vi "dfd_DFXPSimu AccAdd (vector).vi"(5 "quantize output?":bool=TRUE, 7 "op params":T2={"source"=0, "is floating?"=FALSE, "o-mode"=enum."Wrap", "q-mode"=enum."Truncation", "wl"=1, "high limit"=0, "low limit"=0, "iwl"=0, "sign?"=TRUE} {"source" items=["Coef a/k"=0, "Coef b/v"=7, "Input"=1, "Output"=2, "Multiplicand"=3, "Product"=4, "Sum"=5, "Delay"=6, "Gain"=8]}, 8 "filtering statistics in":T6(array[cluster]) {"statistics information"."min value" format="%.2f"; "statistics information"."max value" format="%.2f"; "Quantizer Source" items=["Coefficients a/k"=0, "Coefficients b/v"=7, "Input"=1, "Output"=2, "Multiplicand"=3, "Product"=4, "Sum"=5, "Delay"=6]}, 10 "addends":T7, 11 "acc in":T1={"value"=0, "wl"=0, "iwl"=0, "Signed"=TRUE} {"value" format="%.0x"}) -> (0 "filtering statistics out":T6(array[cluster]) {"statistics information"."min value" format="%.2f"; "statistics information"."max value" format="%.2f"; "Quantizer Source" items=["Coefficients a/k"=0, "Coefficients b/v"=7, "Input"=1, "Output"=2, "Multiplicand"=3, "Product"=4, "Sum"=5, "Delay"=6]}, 3 "acc out":T1={"value"=0, "wl"=0, "iwl"=0, "Signed"=TRUE} {"value" format="%.0x"})   [LabVIEW 2017, in "NI_DigFilter_FXP.lvlib"]
uses:
  <vilib>/addons/Digital Filter Design/NI_DigFilter_FXP.lvlib
  <vilib>/addons/Digital Filter Design/_Objects.llb/dfd_DFXP Data Type (scaler).ctl
  <vilib>/addons/Digital Filter Design/_Objects.llb/dfd_DFXP Data Type (vector).ctl
  <vilib>/addons/Digital Filter Design/_Objects.llb/DFD Quantization Sources.ctl
  <vilib>/addons/Digital Filter Design/_Objects.llb/DFD FXP Statistics Data.ctl
  <vilib>/addons/Digital Filter Design/_Objects.llb/dfd_DFXP Operation Parameter.ctl
  <vilib>/addons/Digital Filter Design/_Objects.llb/dfd_Internal Quantization Srcs.ctl
  <vilib>/addons/Digital Filter Design/NI_DigFilterLicensed.lvlib
panel:
  in  "addend type":T1={"value"=0, "wl"=0, "iwl"=0, "Signed"=TRUE} {"value" format="%.0x"}
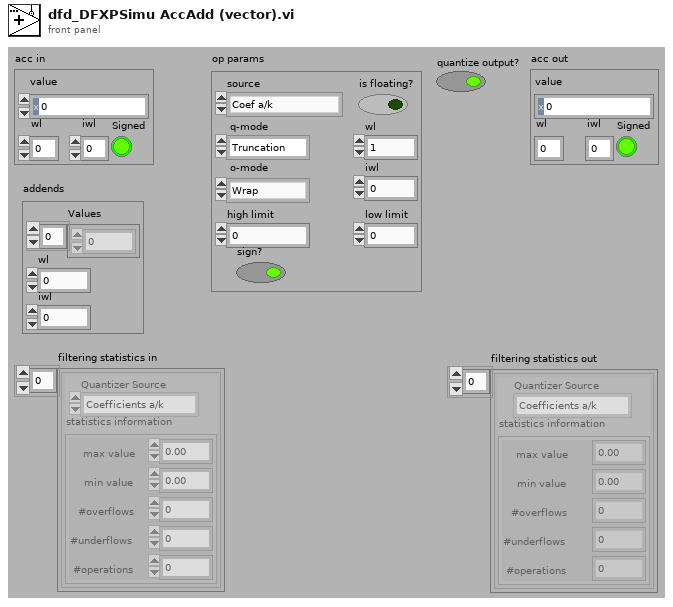
[diagram p1: front panel]
types:
  T1 = typedef "dfd_DFXP Data Type (scaler).ctl" = cluster{"value":i64, "wl":i16, "iwl":i16, "Signed":bool}
  T2 = typedef "dfd_DFXP Operation Parameter.ctl" = cluster{"source":T3, "is floating?":bool, "o-mode":enum16{"Saturation", "Wrap"}, "q-mode":enum16{"Nearest", "Truncation"}, "wl":i16, "high limit":i64, "low limit":i64, "iwl":i16, "sign?":bool}
  T3 = typedef "NI_DigFilterLicensed.lvlib/dfd_Internal Quantization Srcs.ctl" = u16
  T4 = typedef "NI_DigFilterLicensed.lvlib/DFD Quantization Sources.ctl" = u16
  T5 = typedef "NI_DigFilterLicensed.lvlib/DFD FXP Statistics Data.ctl" = cluster{"max value":ext, "min value":ext, "#overflows":i32, "#underflows":i32, "#operations":i32}
  T6 = cluster{"Quantizer Source":T4, "statistics information":T5}[]
  T7 = typedef "dfd_DFXP Data Type (vector).ctl" = cluster{"Values":i64[], "wl":i16, "iwl":i16}
  T8 = cluster{"Quantizer Source":T4, "statistics information":T5}
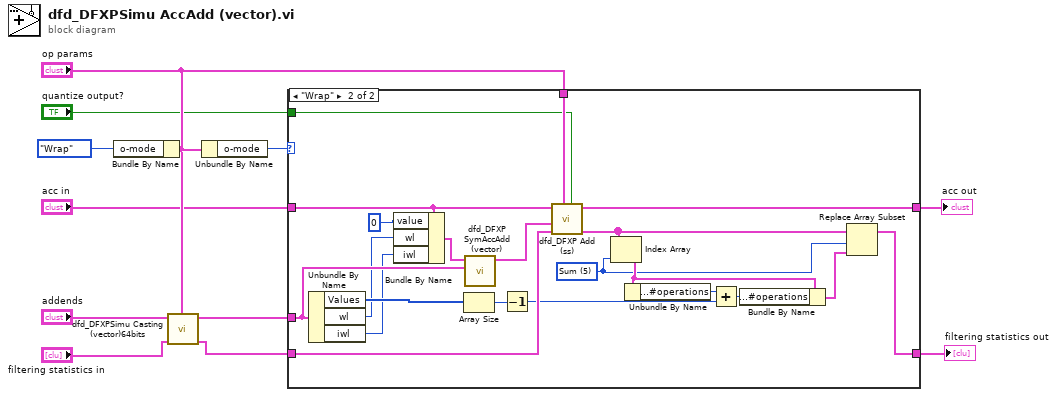
[diagram p0: block diagram]
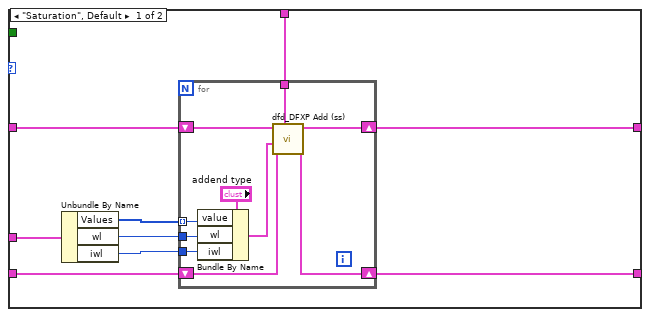
[diagram p2: hidden frame]
diagram:
  n1 = Bundle By Name(cluster="op params", "o-mode"=enum16{"Saturation", "Wrap"}."Wrap" ("o_mode")) -> (w4:T2)
  n2 = call <vilib>:"dfd_DFXPSimu Casting (vector)64bits.vi"("op params"=w4, "filtering statistics in"="filtering statistics in", "Value in"="addends") -> ("filtering statistics out"=w10:T6, "Value out"=w3:T7)  [unwired: 1 in, 6 out]
  n3 = Unbundle By Name("op params") -> ("o-mode"=w6:enum16{"Saturation", "Wrap"})
  n4 = case shown="\"Wrap\"" w6 {
    tunnel: [w21 w51] -> w1
    tunnel: [w20 w40] -> w12
    tunnel: w10 -> [w19 w50]
    tunnel: "op params" -> [w18 w52]
    tunnel: "acc in" -> [w17 w34]
    tunnel: w3 -> [w16 w49]
    tunnel: "quantize output?" -> [_ w32]
    frame "Saturation", Default {
      n5 = Unbundle By Name(w16) -> ("Values"=w15:i64[], "wl"=w14:i16, "iwl"=w13:i16)
      n6 = for {
        tunnel: w18 -> [w28]
        shift-right: [w30] -> w20
        shift-left: w19 -> [w31]
        tunnel: w15 -> [w25] mode=indexing
        shift-right: [w29] -> w21
        shift-left: w17 -> [w27]
        tunnel: w14 -> [w24]
        tunnel: w13 -> [w23]
        n7 = Bundle By Name(cluster="addend type", "value"=w25, "wl"=w24, "iwl"=w23) -> (w22:T1)
        n8 = call <vilib>:"dfd_DFXP Add (ss).vi"("op params"=w28, "filtering statistics in"=w31, "Value in 2"=w22, "Value in"=w27) -> ("filtering statistics out"=w30:T6, "Value out"=w29:T1)  [unwired: 1 in, 5 out]
      }
    }
    frame "Wrap" {
      w43 = T3 5 items=["Coef a/k"=0, "Coef b/v"=7, "Input"=1, "Output"=2, "Multiplicand"=3, "Product"=4, "Sum"=5, "Delay"=6, "Gain"=8] ("source")
      n9 = Unbundle By Name(w49) -> ("Values"=w39:i64[], "wl"=w37:i16, "iwl"=w36:i16)
      n10 = Bundle By Name(cluster=w34, "value"=i64 0, "wl"=w37, "iwl"=w36) -> (w35:T1)
      n11 = Array Size(array=w39) -> (size(s)=w48:i32)
      n12 = call <vilib>:"dfd_DFXP SymAccAdd (vector).vi"("Values in"=w49, "Acc"=w35) -> ("Value out"=w33:T1)  [unwired: 9 out]
      n13 = Decrement(x=w48) -> (x-1=w41:i32)
      n14 = call <vilib>:"dfd_DFXP Add (ss).vi"("quantize output? (T)"=w32, "op params"=w52, "filtering statistics in"=w50, "Value in 2"=w33, "Value in"=w34) -> ("filtering statistics out"=w42:T6, "Value out"=w51:T1)  [unwired: 5 out]
      n15 = Index Array(array=w42, index=w43) -> (element=w45:T8)
      n16 = Unbundle By Name(w45) -> ("statistics information.#operations"=w47:i32)
      n17 = Add(x=w47, y=w41) -> (x+y=w44:i32)
      n18 = Bundle By Name(cluster=w45, "statistics information.#operations"=w44) -> (w46:T8)
      n19 = Replace Array Subset(array=w42, new element=w46, index=w43) -> (w40:T6)
    }
  }
  "filtering statistics out" <- w12
  "acc out" <- w1
